vi "ReadWrite2FIFOs.vi"(0 "ReadBytes":refnum<k21>, 1 "WrittenBytes":refnum<k21>, 2 "Reads":refnum<k21>, 3 "Writes":refnum<k21>, 4 "Port":refnum<k21>) -> ()   [LabVIEW 2023]
uses:
  <vilib>/rvi/Emulation/niFpgaGetClockAttributes.vi
  <vilib>/rvi/Emulation/niFpgaSctlEmulationGetInTimedLoop.vi
  <vilib>/rvi/Emulation/niFpgaEmulationReportErrorSimple.vi
  <vilib>/rvi/DataTransferAndStorage/Container/Common/niFpgaContainerExecOnDevCompGetState.vi
  <vilib>/rvi/Emulation/niFpgaEmulationIsFPGAContextNoSignature.vi
  <vilib>/rvi/errors/niFpgaSetErrorForExecOnDevCompSimple.vi
  <vilib>/rvi/eio/common/nirviEmuReportErrorAndStop.vi
  <vilib>/rvi/DataTransferAndStorage/Container/Common/niFpgaContainerGetUniqueNameForEmu.vi
  <vilib>/rvi/FIFO/Fifo_Resource/nirvififoEmulationSetSize.vi
  <vilib>/rvi/FIFO/Fifo_Resource/nirviFifoEmulationQueueMgr.vi
  <instcachedir>/0/nirviFifoEmulationQueueMgr_E5CAEC123FF24DC58D834DCA3CDAA9B5.lvgen/nirviFifoEmulationQueueMgr_E5CAEC123FF24DC58D834DCA3CDAA9B5_002.vi
  <vilib>/rvi/FIFO/Fifo_Resource/nirvififoEmulationDetermineInputValidOut.vi
  <vilib>/rvi/FIFO/Fifo_Resource/nirvififoEmulationCreateLock.vi
  <vilib>/rvi/Emulation/niFpgaProcessEmulError.vi
  <vilib>/rvi/FIFO/Fifo_Resource/nirvififoEmulationObtainLock.vi
  <vilib>/rvi/FIFO/Fifo_Resource/nirvififoEmulationReleaseLock.vi
  <vilib>/rvi/occurrence/nirviWaitOnOccurrenceBase.vi
  <vilib>/rvi/errors/nirviReportUnexpectedCaseInternalError.vi
  <vilib>/rvi/errors/nirviReportUnexpectedCaseInternalError (U32).vi
  <vilib>/Utility/error.llb/Clear Errors.vi
  <vilib>/eio/utilities/niEioResolveVilibRelativePath.vi
  <vilib>/rvi/interface/RandomDataEmulation/niFpgaRandomDataHandleErrors.vi
  <vilib>/rvi/eio/common/nirviEmuTemplateMethod_errors.vi
  <vilib>/rvi/Memory/Memory_Emulation/niFpgaMemoryEmulationCacheClearOnFirstRun.vi
  <vilib>/rvi/Memory/Memory_Emulation/nirvimemoryEmulationManagerCache_MakeExclusive.vi
  <vilib>/rvi/Memory/Memory_Emulation/niFpgaMemoryEmulationValidateCache.vi
  <vilib>/rvi/Memory/Memory_Emulation/nirvimemoryEmulationManagerCache_InsertValue.vi
  <vilib>/rvi/Memory/Memory_Emulation/nirvimemoryEmulationManagerCache_ReleaseExclusive.vi
  <vilib>/rvi/Memory/Memory_Emulation/nirvimemoryEmulationManagerCache_GetValue.vi
  <vilib>/rvi/Memory/Memory_Emulation/nirvimemoryEmulationManagerCache_SetValue.vi
  <vilib>/rvi/Emulation/niFpgaCriticalErrorInLSC.vi
  <vilib>/rvi/DataTransferAndStorage/Container/XNode/niFpgaContainer.xnode
  <vilib>/rvi/FIFO/Fifo_Resource/niFpgaFifoEmulationRefIn.vi
  <vilib>/eio/EIOMethodNode/EIOMethodNode.xnode
  <vilib>/rvi/DataTransferAndStorage/Register/Emulation/niFpgaRegisterEmulationRefIn.vi
panel:
  # "Copy data from Writes FIFO into port, output\ndata on Reads FIFO. Just an interface on top of serial port."
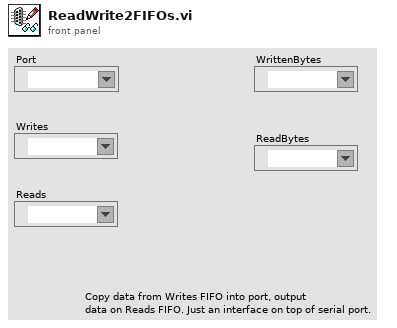
[diagram p1: front panel]
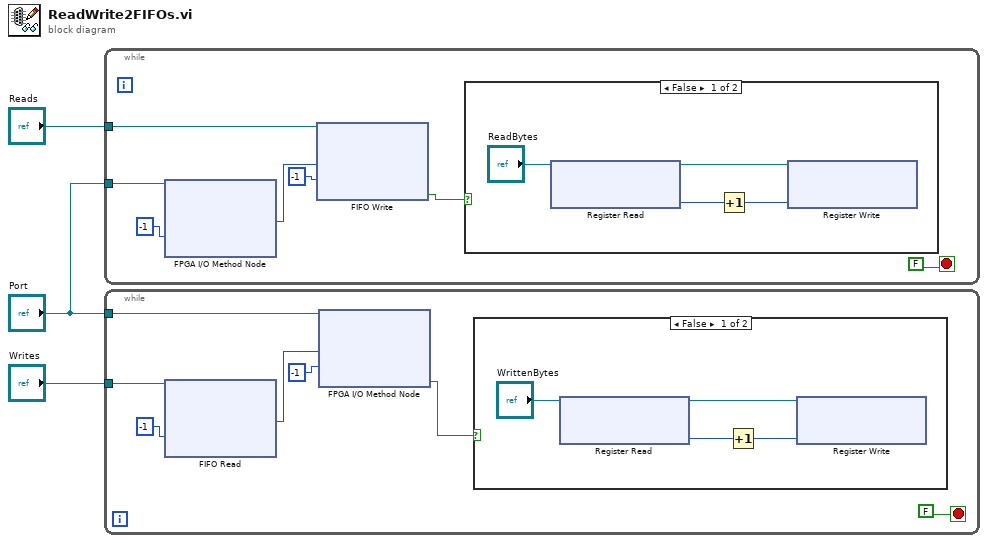
[diagram p0: block diagram]
diagram:
  n1 = while {
    tunnel: "Port" -> [w9]
    tunnel: "Reads" -> [w7]
    stop <- FALSE stop-if-true
    n2 = xnode "FPGA I/O Method Node"("FPGA I/O In"=w9, "Timeout (ms)"=-1) -> ("Data"=w5:u8)  [unwired: 2 out]
    n3 = xnode ("FIFO Write")("Element"=w5, "Timeout"=-1, "FIFO In"=w7) -> ("Timed Out?"=w4:bool)  [unwired: 1 out]
    n4 = case shown="False" w4 {
      frame False {
        n5 = xnode ("Register Read")("Register In"="ReadBytes") -> ("Data"=w13:u32, "Register Out"=w12:refnum<k21>)
        n6 = Increment(x=w13) -> (x+1=w11:u32)
        n7 = xnode ("Register Write")("Data"=w11, "Register In"=w12) -> ()  [unwired: 1 out]
      }
      frame True {
      }
    }
  }
  n8 = while {
    tunnel: "Port" -> [w16]
    tunnel: "Writes" -> [w17]
    stop <- FALSE stop-if-true
    n9 = xnode ("FIFO Read")("Timeout"=-1, "FIFO In"=w17) -> ("Element"=w18:u8)  [unwired: 2 out]
    n10 = xnode "FPGA I/O Method Node"("FPGA I/O In"=w16, "Data"=w18, "Timeout (ms)"=-1) -> ("Timed Out"=w15:bool)  [unwired: 1 out]
    n11 = case shown="False" w15 {
      frame False {
        n12 = xnode ("Register Read")("Register In"="WrittenBytes") -> ("Data"=w24:u32, "Register Out"=w23:refnum<k21>)
        n13 = Increment(x=w24) -> (x+1=w22:u32)
        n14 = xnode ("Register Write")("Data"=w22, "Register In"=w23) -> ()  [unwired: 1 out]
      }
      frame True {
      }
    }
  }
